vi "Acquire Joint Positions.vi"() -> ()   [LabVIEW 2011, in "KinectOne.lvlib"]
doc: "This example demonstrates how to track joint positions using the Kinect One."
uses:
  vi.lib/MakerHub/KinectOne/KinectOne.lvlib
  vi.lib/MakerHub/KinectOne/Private/Type Defs/JointType.ctl
  vi.lib/MakerHub/KinectOne/Private/Type Defs/Joint Position.ctl
  vi.lib/MakerHub/KinectOne/Private/Initialize Image [Color].vi
  vi.lib/MakerHub/KinectOne/Private/kinectRead [BodyFrame].vi
  Microsoft.Kinect
  C:/github/makerhub/KinectOne/LabVIEW/vi.lib/MakerHub/KinectOne/Private/Libs/BodyFrameDataInterface.dll
  vi.lib/MakerHub/KinectOne/Private/Libs/BodyFrameDataInterface.dll
panel:
  out "Joint Position":T1
  in  "JointType":T2=enum."Head"
  out "Body Index Image":T3(plugin-control)
  in  "Stop Button":bool
  # "Acquire Joint Position Example\n\nThis example demonstrates how to acquire color images from the Kinect One.\n\n1. Make sure you have the Kinect SDK 2.0 installed.\n2. Connect the Kinect sensor to the computer via USB.\n3. Click the Run button.\n4. Stand in front of the Kinect sensor.\n\nHave feedback or need help?  Visit the MakerHub forums at www.labviewmakerhub.com/forums/kinectone"
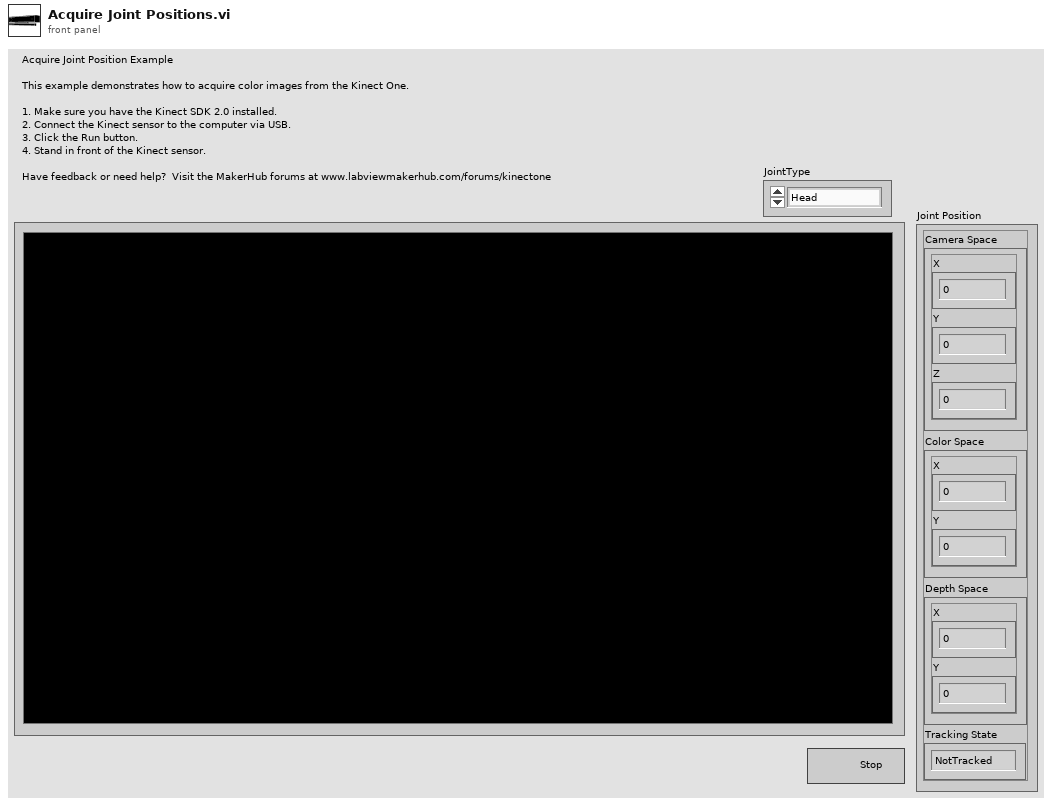
[diagram p1: front panel]
types:
  T1 = typedef "KinectOne.lvlib/Joint Position.ctl" = cluster{"Camera Space":cluster{"X":dbl, "Y":dbl, "Z":dbl}, "Color Space":cluster{"X":dbl, "Y":dbl}, "Depth Space":cluster{"X":dbl, "Y":dbl}, "Tracking State":enum16{"NotTracked", "Inferred", "Tracked"}}
  T2 = typedef "KinectOne.lvlib/JointType.ctl" = enum16{"SpineBase", "SpineMid", "Neck", "Head", "ShoulderLeft", "ElbowLeft", "WristLeft", "HandLeft", "ShoulderRight", "ElbowRight", "WristRight", "HandRight", "HipLeft", "KneeLeft", "AnkleLeft", "FootLeft", "HipRight", "KneeRight", "AnkleRight", "FootRight", "SpineShoulder", "HandTipLeft", "ThumbLeft", "HandTipRight", "ThumbRight"}
  T3 = typedef "IMAQ Image.ctl" = refnum<image>
  T4 = typedef "KinectOne.lvlib/KinectSensor References.ctl" = cluster{"KinectSensor":refnum<k24>, "MultiSourceFrameReader":refnum<k24>, "BodyFrameDataInterface":refnum<k24>}
  T5 = typedef "KinectOne.lvlib/BodyData.ctl" = cluster{"ClippedEdges":T6, "HandLeftConfidence":T7, "HandLeftState":T8, "HandRightConfidence":T9, "HandRightState":T10, "IsRestricted":bool, "IsTracked":bool, "JointOrientations":refnum<k24>, "Joints":refnum<k24>, "Lean":refnum<k24>, "LeanTrackingState":T11, "TrackingId":u64}
  T6 = typedef "KinectOne.lvlib/ClippedEdges.ctl" = enum16{"None", "Right", "Left", "Top", "Bottom"}
  T7 = typedef "KinectOne.lvlib/HandLeftConfidence.ctl" = enum16{"Low", "High"}
  T8 = typedef "KinectOne.lvlib/HandLeftState.ctl" = enum16{"Unknown", "NotTracked", "Open", "Closed", "Lasso"}
  T9 = typedef "KinectOne.lvlib/HandRightConfidence.ctl" = enum16{"Low", "High"}
  T10 = typedef "KinectOne.lvlib/HandRightState.ctl" = enum16{"Unknown", "NotTracked", "Open", "Closed", "Lasso"}
  T11 = typedef "KinectOne.lvlib/LeanTrackingState.ctl" = enum16{"NotTracked", "Inferred", "Tracked"}
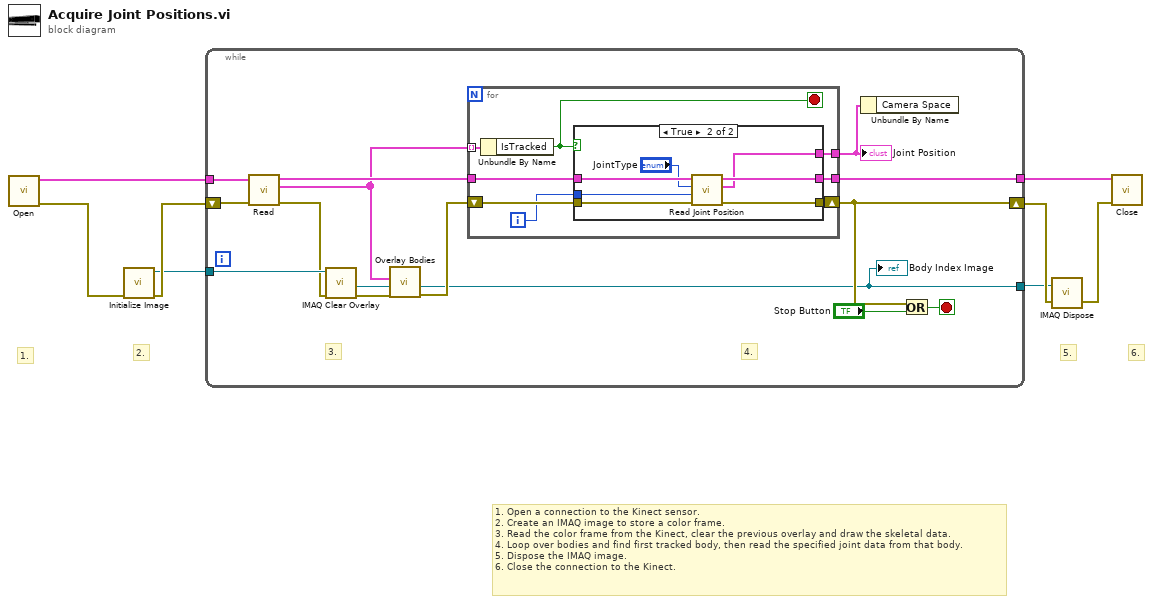
[diagram p0: block diagram]
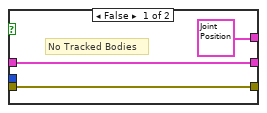
[diagram p2: hidden frame]
diagram:
  # "1. Open a connection to the Kinect sensor.\n2. Create an IMAQ image to store a color frame.\n3. Read the color frame from the Kinect, clear the previous overlay and draw the skeletal data.\n4. Loop over bodies and find first tracked body, then read the specified joint data from that body.\n5. Dispose the IMAQ image.\n6. Close the connection to the Kinect."
  # "6."
  # "5."
  # "2."
  # "1."
  n1 = call "Open.vi"() -> ("Error Out"=w7:errorcluster, "KinectSensor References out"=w3:T4)  [unwired: 10 in]
  n2 = call-poly "Initialize Image.vi"("Error In"=w7) -> ("Error Out"=w2:errorcluster, "Color Image"=w1:T3)  [unwired: 9 in]
  n3 = while {
    shift-right: [w15] -> w6
    shift-left: w2 -> [w17]
    tunnel: [w10] -> w5
    tunnel: [w13] -> w4
    tunnel: w3 -> [w14]
    tunnel: w1 -> [w21]
    stop <- w23 stop-if-true
    # "4."
    # "3."
    n4 = call-poly "Read.vi"("error in (no error)"=w17, "KinectSensor References in"=w14) -> ("error out"=w19:errorcluster, "Body Data"=w11:T5[], "KinectSensor References out"=w12:T4)  [unwired: 7 in]
    n5 = call "IMAQ Clear Overlay"("error in (no error)"=w19, "Image"=w21) -> ("error out"=w18:errorcluster, "Image Out"=w20:T3)  [unwired: 8 in]
    n6 = call "Overlay Bodies.vi"("Error In"=w18, "Image"=w20, "Body Data"=w11) -> ("Error Out"=w16:errorcluster, "Image Out"=w10:T3)  [unwired: 7 in]
    "Body Index Image" <- w10
    n7 = for {
      tunnel: [w29] -> w13
      tunnel: w12 -> [w28]
      tunnel: [w27] -> w9
      shift-right: [w30] -> w15
      shift-left: w16 -> [w31]
      tunnel: w11 -> [w26] mode=indexing
      i -> [w24]
      stop <- w25 stop-if-true
      n8 = Unbundle By Name(w26) -> ("IsTracked"=w25:bool)
      n9 = case shown="True" w25 {
        tunnel: w31 -> [w33 w41]
        tunnel: [w33 w40] -> w30
        tunnel: [w34 w39] -> w29
        tunnel: w28 -> [w34 w38]
        tunnel: [T1 {"Camera Space"={"X"=0.0, "Y"=0.0, "Z"=0.0}, "Color Space"={"X"=0.0, "Y"=0.0}, "Depth Space"={"X"=0.0, "Y"=0.0}, "Tracking State"=enum."NotTracked"} ("Joint Position") w36] -> w27
        tunnel: w24 -> [_ w35]
        frame False {
          # "No Tracked Bodies"
        }
        frame True {
          n10 = call "Read Joint Position.vi"("Error In"=w41, "Body Index"=w35, "JointType"="JointType", "KinectSensor References"=w38) -> ("Error Out"=w40:errorcluster, "Joint Position"=w36:T1, "KinectSensor References"=w39:T4)  [unwired: 4 in, 1 out]
        }
      }
    }
    "Joint Position" <- w9
    n11 = Unbundle By Name(w9) -> ()  [unwired: 1 out]
    n12 = Or(x=w15, y="Stop Button") -> (x .or. y?=w23:bool)
  }
  n13 = call "IMAQ Dispose"("Image"=w5, "error in (no error)"=w6) -> ("error out"=w8:errorcluster)  [unwired: 4 in]
  n14 = call "Close.vi"("Error In"=w8, "KinectSensor References"=w4) -> ()  [unwired: 9 in, 1 out]
